vi "sub_FFT normalizado positivo.vi"(9 "FFT size":i32, 10 "Array in":dbl[](array[numeric]), 11 "WaveformGraph in":refnum<vi>) -> (3 "Array out":dbl[](array[numeric]))   [LabVIEW 2020]
uses:
  <vilib>/Analysis/2dsp.llb/Real FFT.vi
  <vilib>/Analysis/NI_AALPro.lvlib
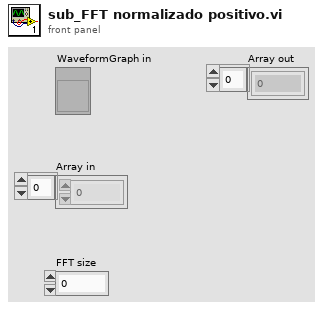
[diagram p1: front panel]
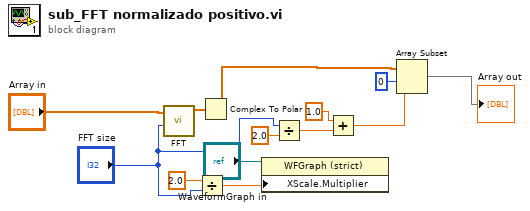
[diagram p0: block diagram]
diagram:
  n1 = call-poly <vilib>:"FFT.vi"("FFT size"="FFT size", "X"="Array in") -> ("FFT {X}"=w2:cdb[])  [unwired: 8 in, 1 out]
  n2 = Divide(x=2.0, y="FFT size") -> (x/y=w4:dbl)
  n3 = Complex To Polar(r * e^(i*theta)=w2) -> (r=w6:dbl[])  [unwired: 1 out]
  n4 = property on="Property Node" class="WFGraph (strict)"(reference="WaveformGraph in", "XScale.Multiplier"=w4) -> ()  [unwired: 1 in, 2 out]
  n5 = Divide(x="FFT size", y=2.0 ("x")) -> (x/y=w10:dbl)
  n6 = Add(x=1.0, y=w10) -> (x+y=w11:dbl)
  n7 = Array Subset(array=w6, index=0, length=w11) -> (→"Array out":dbl[])
